vi "Set Start Trigger (Formula).vi"(5 "Retriggerable (F)":bool, 7 "Pre-Trigger Duration (0 s)":dbl, 8 "error in (no error)":errorcluster, 9 "Variable Mappings":T2[](array[typedef]), 10 "Trigger Condition":string, 11 "Data Logging Specification Ref in":T1) -> (0 "error out":errorcluster, 3 "Data Logging Specification Ref out":T1)   [LabVIEW 2020, in "NI_VS Data Logging API.lvlib"]
doc: "Specifies a trigger condition on which to stop logging data. You also can specify whether to continue logging channel data for a set period of time after the trigger condition occurs.\n\nYou must manually select the polymorphic instance to use."
uses:
  <vilib>/NI VeriStand/Execution/DataLogging/NI_VS Data Logging API.lvlib
  <vilib>/NI VeriStand/Execution/DataLogging/DataLoggingSpecification Ref.ctl
  NationalInstruments.VeriStand.ClientAPI
  <vilib>/NI VeriStand/Execution/DataLogging/Variable Mapping.ctl
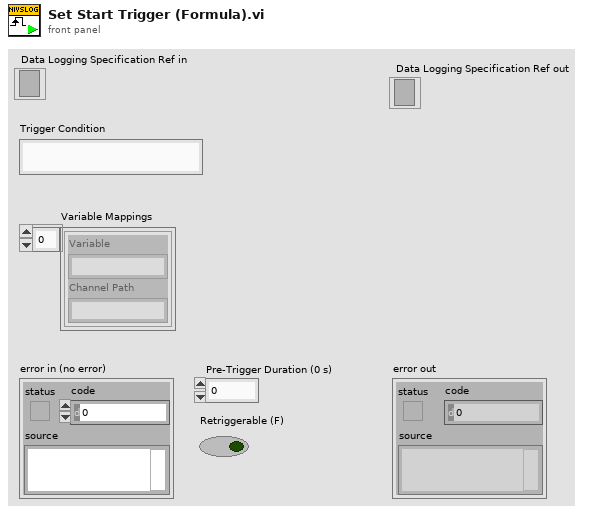
[diagram p1: front panel]
types:
  T1 = typedef "NI_VS Data Logging API.lvlib/DataLoggingSpecification Ref.ctl" = refnum<k24>
  T2 = typedef "NI_VS Data Logging API.lvlib/Variable Mapping.ctl" = cluster{"Variable":string, "Channel Path":string}
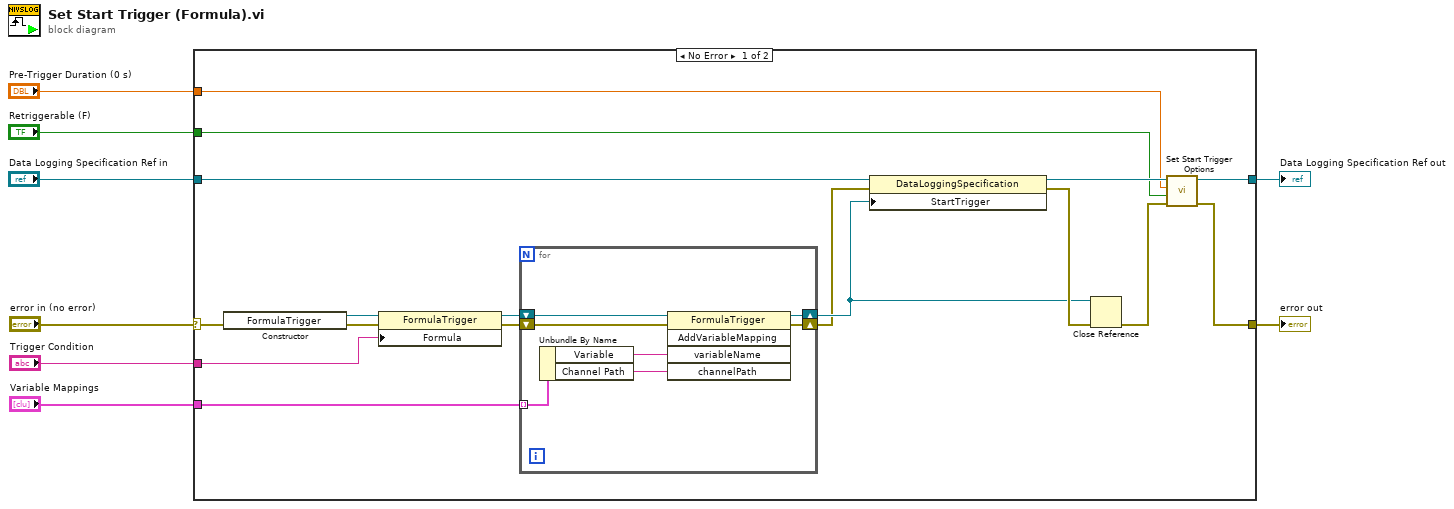
[diagram p0: block diagram]
diagram:
  n1 = case shown="No Error" "error in (no error)" {
    selector: "error in (no error)" -> [w15 w34]
    tunnel: "Variable Mappings" -> [w14 _]
    tunnel: "Trigger Condition" -> [w13 _]
    tunnel: "Data Logging Specification Ref in" -> [w24 w33]
    tunnel: [w21 w33] -> w5
    tunnel: [w20 w34] -> w4
    tunnel: "Pre-Trigger Duration (0 s)" -> [w10 _]
    tunnel: "Retriggerable (F)" -> [w9 _]
    frame No Error {
      n2 = constructor class="FormulaTrigger"(error in=w15) -> (reference out=w19:refnum<k24>, error out=w18:errorcluster)  [unwired: 2 in, 1 out]
      n3 = property class="FormulaTrigger"(reference=w19, error in=w18, "Formula"=w13) -> (reference out=w17:refnum<k24>, error out=w16:errorcluster)
      n4 = for {
        shift-right: [w30] -> w12
        shift-left: w17 -> [w32]
        shift-right: [w29] -> w11
        shift-left: w16 -> [w31]
        tunnel: w14 -> [w28] mode=indexing
        n5 = Unbundle By Name(w28) -> ("Variable"=w27:string, "Channel Path"=w26:string)
        n6 = invoke class="FormulaTrigger" method="AddVariableMapping"(reference=w32, error in=w31, "variableName"=w27, "channelPath"=w26) -> (reference out=w30:refnum<k24>, error out=w29:errorcluster)  [unwired: 1 in, 3 out]
      }
      n7 = property class="DataLoggingSpecification"(reference=w24, error in=w11, "StartTrigger"=w12) -> (reference out=w23:T1, error out=w25:errorcluster)
      n8 = Close Reference(reference=w12, error in (no error)=w25) -> (error out=w22:errorcluster)
      n9 = call <vilib>:"Set Start Trigger Options.vi"("error in (no error)"=w22, "Retriggerable"=w9, "Pre-Trigger Duration"=w10, "Data Logging Specification Ref in"=w23) -> ("error out"=w20:errorcluster, "Data Logging Specification Ref out"=w21:T1)  [unwired: 6 in]
    }
    frame Error {
    }
  }
  "error out" <- w4
  "Data Logging Specification Ref out" <- w5
